vi "write_to_file.vi"(0 "refnum":refnum<file>, 1 "Time":dbl, 5 "y data":dbl, 7 "y data precision":i16, 9 "x data":dbl, 11 "x data precision":i16, 12 "Setpoint":dbl) -> (4 "dup refnum":refnum<file>)   [LabVIEW 2012]
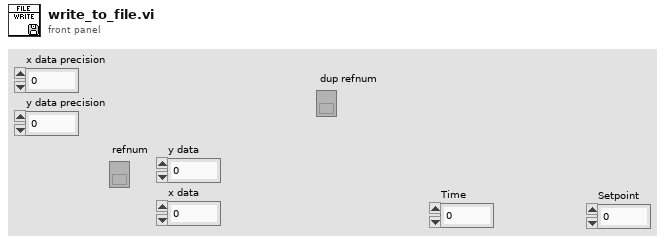
[diagram p1: front panel]
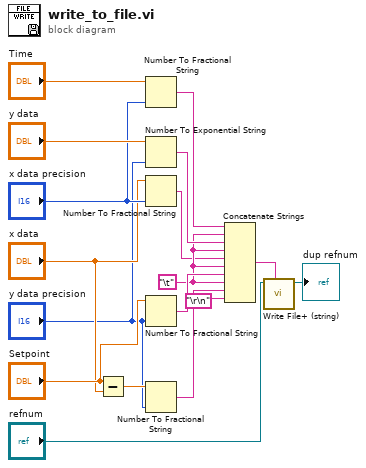
[diagram p0: block diagram]
diagram:
  w8 = "\t"
  n1 = Subtract(x="Setpoint", y="x data") -> (x-y=w5:dbl)
  n2 = Number To Fractional String(number="Time", precision (6)="x data precision") -> (F-format string=w2:string)  [unwired: 2 in]
  n3 = Number To Exponential String(number="y data", precision (6)="y data precision") -> (E-format string=w16:string)  [unwired: 2 in]
  n4 = Number To Fractional String(number="x data", precision (6)="x data precision") -> (F-format string=w1:string)  [unwired: 2 in]
  n5 = Number To Fractional String(number="Setpoint", precision (6)="y data precision") -> (F-format string=w12:string)  [unwired: 2 in]
  n6 = Number To Fractional String(number=w5, precision (6)="y data precision") -> (F-format string=w3:string)  [unwired: 2 in]
  n7 = Concatenate Strings(w2, w8, w16, w8, w1, w8, w12, w8, w3, "\r\n") -> (w17:string)
  n8 = call <vilib>:"Write File+ (string).vi"("string"=w17, "refnum"="refnum") -> ("dup refnum"=→"dup refnum":refnum<file>)  [unwired: 5 in, 2 out]
